vi "Tick Count (U64) Engine.vi"() -> ()   [LabVIEW 2015]
uses:
  <vilib>/Platform/TimedLoop/XDataNode/timing_clust.ctl
  <vilib>/Platform/TimedLoop/XDataNode/nitl_modes.ctl
  <vilib>/Platform/TimedLoop/XDataNode/wakeup.ctl
  <vilib>/rvi/Emulation/niFpgaSctlEmulationGetInTimedLoop.vi
  <vilib>/rvi/Emulation/niFpgaEmulationReportErrorSimple.vi
  <vilib>/rvi/Emulation/niFpgaGetClockAttributes.vi
  <vilib>/rvi/Emulation/niFpgaCriticalErrorInLSC.vi
  <vilib>/rvi/Emulation/niFpgaProcessEmulError.vi
  Tick Count (U64) Global.vi
  <vilib>/Platform/TimedLoop/XDataNode/XDataNode.xnode
  <vilib>/rvi/Arithmetic/AddSubMult/XNode/nirviSatArithmetic.xnode
  <vilib>/Platform/TimedLoop/XDataNode/XDNodeRunTimeDep.lvlib
panel:
  out "Tick Count (U64)":u64
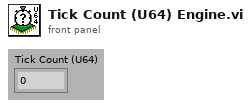
[diagram p1: front panel]
types:
  T1 = typedef "XDNodeRunTimeDep.lvlib/timing_clust.ctl" = cluster{"Expected End [f-1]":u64, "Actual End [f-1]":u64, "Finished Late? [f-1]":bool, "Expected End [i-1]":u64, "Actual End [i-1]":u64, "Finished Late? [i-1]":bool, "Expected Start [i]":u64, "Actual Start [i]":u64, "Expected Start [f]":u64, "Actual Start [f]":u64, "Source Name":string, "Structure Name":string, "Period":i64, "Deadline":i64, "Offset":i64, "Start":i64, "Priority":i32, "Timeout":i32, "Mode":T2, "Wakeup Reason":T3, "Error":errorcluster, "Source Type":string, "Secondary Source Type":string, "Global End Time":u64, "Global Start Time":u64, "Frame Duration":u64, "Iteration Duration":u64, "Assigned CPU":i32, "I/O Scan Engine Mode":u32}
  T2 = typedef "XDNodeRunTimeDep.lvlib/nitl_modes.ctl" = enum32{"No Change", "Process missed periods, maintain original phase", "Discard missed periods, maintain original phase", "Process missed periods, ignore original phase", "Discard missed periods, ignore original phase"}
  T3 = typedef "XDNodeRunTimeDep.lvlib/wakeup.ctl" = enum32{"Normal", "Aborted", "Asynchronous wakeup", "Timing source error", "Timed loop error", "Timeout"}
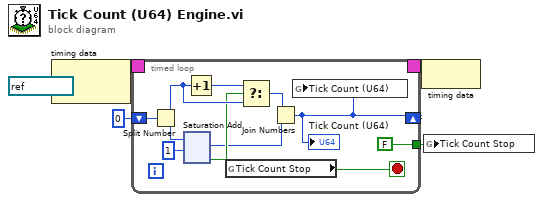
[diagram p0: block diagram]
diagram:
  n1 = node-c288(refnum<k21> "80MHz" ("소스 이름")) -> (w5:T1)
  n2 = timed-loop {
    timing: w5 -> [_]
    timing-out: [_] -> w4
    shift-right: [w8] -> _
    shift-left: u64 0 -> [w16]
    tunnel: [FALSE] -> w2
    stop <- w7 stop-if-true
    n3 = Split Number(x=w16) -> (hi(x)=w13:u32, lo(x)=w15:u32)
    n4 = xnode "Saturation Add"("x"=w15, "y"=u32 1) -> ("x+y"=w9:u32, "overflow"=w10:bool)
    n5 = Increment(x=w13) -> (x+1=w14:u32)
    n6 = global read "Tick Count (U64) Global.vi" "Tick Count Stop"() -> (w7:bool)
    n7 = Select(t=w14, s=w10, f=w13) -> (s? t:f=w12:u32)
    n8 = Join Numbers(hi=w12, lo=w9) -> ((hi.lo)=w8:u64)
    "Tick Count (U64)" <- w8
    n9 = global write "Tick Count (U64) Global.vi" "Tick Count (U64)"(w8) -> ()
  }
  n10 = node-c288(w4) -> ()
  n11 = global write "Tick Count (U64) Global.vi" "Tick Count Stop"(w2) -> ()
